vi "Process Data.vi"(7 "AdasLvTemplate in":refnum<class "AdasLvTemplate.lvclass">, 8 "error in":errorcluster, 11 "Node in":refnum<class "BLS Power Supply Template.lvclass">) -> (0 "error out":errorcluster, 3 "Node out":refnum<class "BLS Power Supply Template.lvclass">, 5 "AdasLvTemplate out":refnum<class "AdasLvTemplate.lvclass">)   [LabVIEW 2023, in "BLS Power Supply Template.lvlib" / "BLS Power Supply Template.lvclass"]
uses:
  BLS Power Supply Template.lvclass
  BLS Power Supply Template.lvclass/BLS Power Supply Template.ctl
  bls-capabilities/src/Capabilities/High Level Capabilities/Power Supply/Power Supply.lvclass
  bls-capabilities/src/Capabilities/High Level Capabilities/Power Supply/Voltage Read Single.vi
  bls-capabilities/src/Capabilities/High Level Capabilities/Power Supply/Output Enable Read Single.vi
  bls-capabilities/src/Capabilities/High Level Capabilities/Power Supply/Current Read Single.vi
  bls-capabilities/src/Capabilities/High Level Capabilities/Power Supply/Voltage Max Read Single.vi
  bls-capabilities/src/Capabilities/High Level Capabilities/Power Supply/Voltage Min Read Single.vi
  bls-capabilities/src/Capabilities/High Level Capabilities/Power Supply/Current Max Read Single.vi
  bls-capabilities/src/Capabilities/High Level Capabilities/Power Supply/Current Min Read Single.vi
  bls-capabilities/src/Capabilities/High Level Capabilities/Power Supply/Power Max Read Single.vi
  bls-capabilities/src/Capabilities/High Level Capabilities/Power Supply/Power Min Read Single.vi
  bls-capabilities/src/Capabilities/High Level Capabilities/Power Supply/Voltage Grad Read Single.vi
  bls-capabilities/src/Capabilities/High Level Capabilities/Power Supply/Power Read Single.vi
  bls-capabilities/src/Capabilities/High Level Capabilities/Power Supply/Power Grad Read Single.vi
  bls-capabilities/src/Capabilities/High Level Capabilities/Power Supply/Current Grad Read Single.vi
  bls-capabilities/src/Capabilities/High Level Capabilities/Power Supply/Control Mode Read Single.vi
  bls-capabilities/src/Capabilities/High Level Capabilities/Power Supply/Error Channels Write Single.vi
  bls-capabilities/src/Capabilities/High Level Capabilities/Power Supply/Control Mode Write Single.vi
  bls-capabilities/src/Capabilities/High Level Capabilities/Power Supply/Power Write Single.vi
  bls-capabilities/src/Capabilities/High Level Capabilities/Power Supply/Current Write Single.vi
  bls-capabilities/src/Capabilities/High Level Capabilities/Power Supply/Output Enable Write Single.vi
  bls-capabilities/src/Capabilities/High Level Capabilities/Power Supply/Voltage Write Single.vi
  <vilib>/ADAS Replay HIL/ADAS Plugin Utilities/AdasLvTemplate/AdasLvTemplate.lvclass
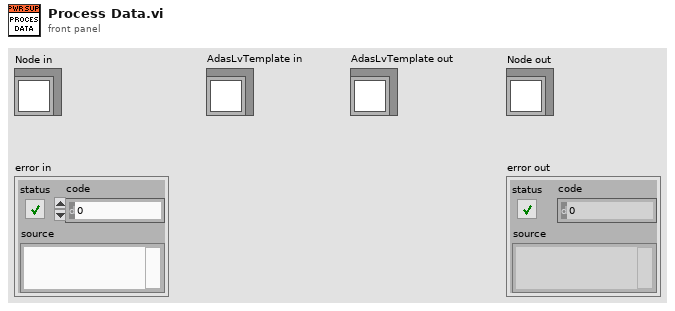
[diagram p1: front panel]
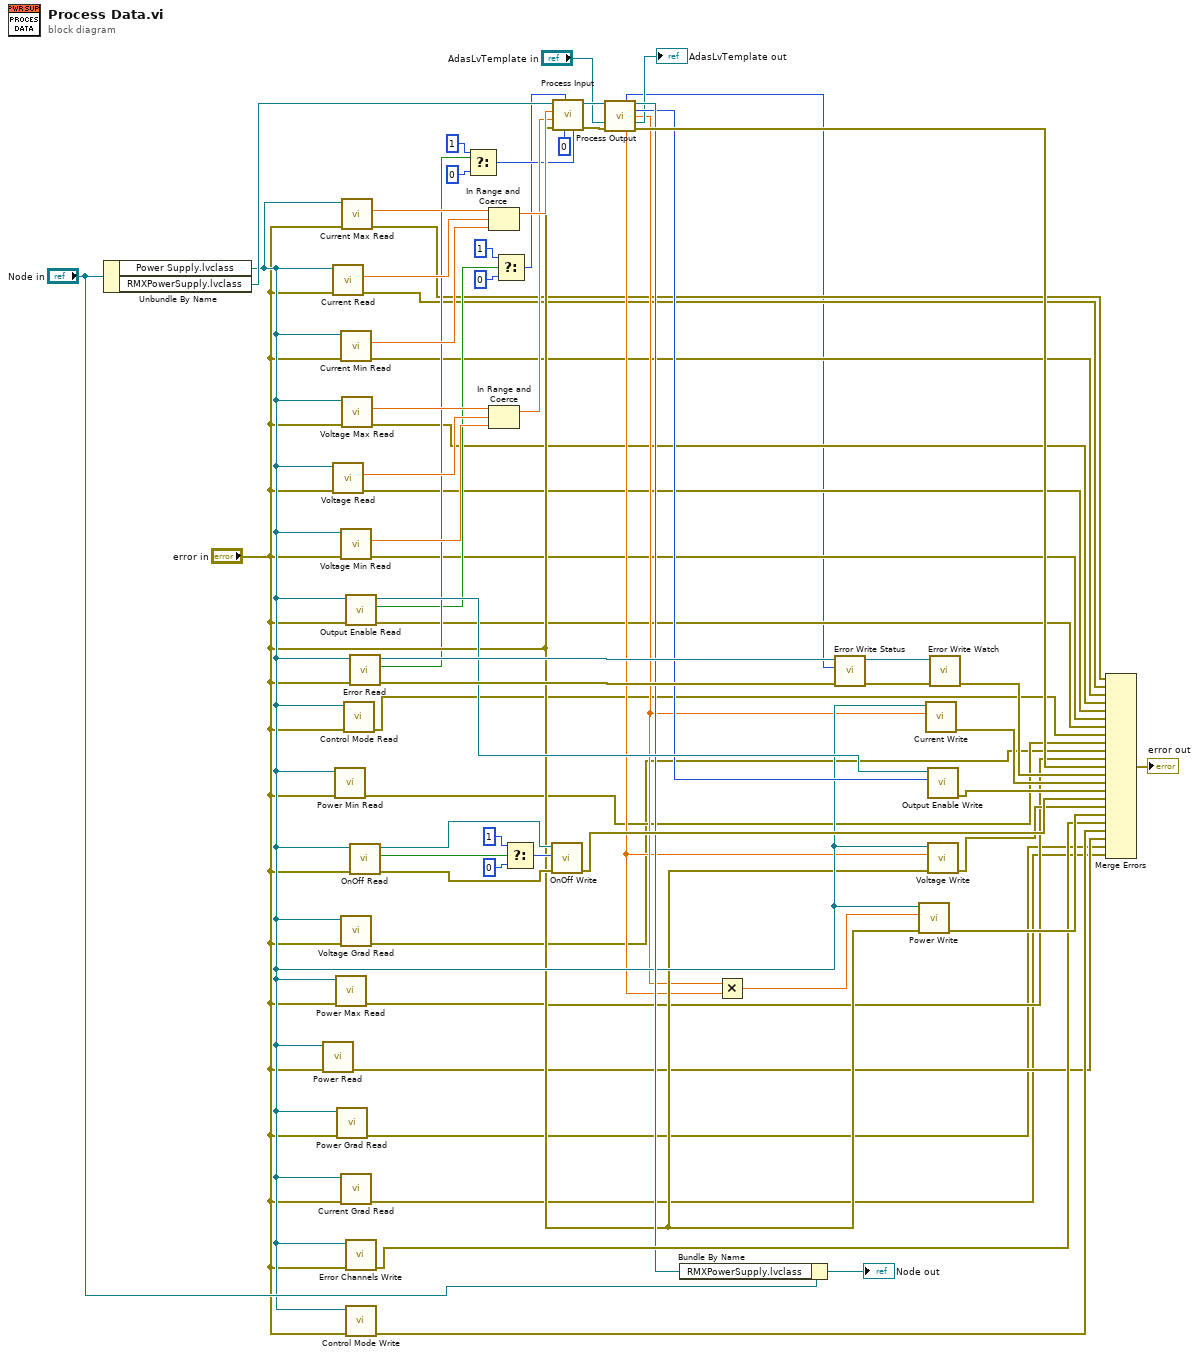
[diagram p0: block diagram]
diagram:
  n1 = Unbundle By Name("Node in") -> ("Power Supply.lvclass"=w28:refnum<class "Power Supply.lvclass">, "RMXPowerSupply.lvclass"=w54:refnum<class "RMXPowerSupply.lvclass">)
  n2 = call-poly "Power Read.vi"("error in"="error in", "Power Supply In"=w28) -> ("error out"=w5:errorcluster)  [unwired: 6 in, 3 out]
  n3 = call-poly "Current Read.vi"("error in"="error in", "Power Supply In"=w28) -> ("error out"=w15:errorcluster, "Current SP"=w38:dbl)  [unwired: 6 in, 2 out]
  n4 = call-poly "Voltage Read.vi"("error in"="error in", "Power Supply In"=w28) -> ("error out"=w12:errorcluster, "Voltage SP"=w43:dbl)  [unwired: 6 in, 2 out]
  n5 = call-poly "Power Min Read.vi"("error in"="error in", "Power Supply In"=w28) -> ("error out"=w8:errorcluster)  [unwired: 6 in, 3 out]
  n6 = call-poly "Power Max Read.vi"("error in"="error in", "Power Supply In"=w28) -> ("error out"=w6:errorcluster)  [unwired: 6 in, 3 out]
  n7 = call-poly "Power Grad Read.vi"("error in"="error in", "Power Supply In"=w28) -> ("error out"=w4:errorcluster)  [unwired: 6 in, 3 out]
  n8 = call-poly "Current Min Read.vi"("error in"="error in", "Power Supply In"=w28) -> ("error out"=w14:errorcluster, "Current Min SP"=w39:dbl)  [unwired: 6 in, 2 out]
  n9 = call-poly "Voltage Min Read.vi"("error in"="error in", "Power Supply In"=w28) -> ("error out"=w11:errorcluster, "Voltage Min SP"=w45:dbl)  [unwired: 6 in, 2 out]
  n10 = call-poly "Voltage Grad Read.vi"("error in"="error in", "Power Supply In"=w28) -> ("error out"=w7:errorcluster)  [unwired: 6 in, 3 out]
  n11 = call-poly "Current Grad Read.vi"("error in"="error in", "Power Supply In"=w28) -> ("error out"=w3:errorcluster)  [unwired: 6 in, 3 out]
  n12 = call-poly "Current Max Read.vi"("error in"="error in", "Power Supply In"=w28) -> ("error out"=w16:errorcluster, "Current Max SP"=w40:dbl)  [unwired: 6 in, 2 out]
  n13 = call-poly "Voltage Max Read.vi"("error in"="error in", "Power Supply In"=w28) -> ("error out"=w13:errorcluster, "Voltage Max SP"=w44:dbl)  [unwired: 6 in, 2 out]
  n14 = call-poly "Control Mode Read.vi"("error in"="error in", "Power Supply In"=w28) -> ("error out"=w9:errorcluster)  [unwired: 6 in, 3 out]
  n15 = call-poly "Output Enable Read.vi"("error in"="error in", "Power Supply In"=w28) -> ("error out"=w10:errorcluster, "Output Enable ACT"=w20:bool, "Power Supply Out"=w35:refnum<class "Power Supply.lvclass">)  [unwired: 6 in, 1 out]
  n16 = call-poly "Error Channels Write.vi"("error in"="error in", "Power Supply In"=w28) -> ("error out"=w58:errorcluster)  [unwired: 8 in, 1 out]
  n17 = call-poly "Control Mode Write.vi"("error in"="error in", "Power Supply In"=w28) -> ("error out"=w57:errorcluster)  [unwired: 8 in, 1 out]
  n18 = call "Error Read.vi"("error in"="error in", "Power Supply In"=w28) -> ("error out"=w42:errorcluster, "Error ACT"=w24:bool, "Power Supply Out"=w41:refnum<class "Power Supply.lvclass">)  [unwired: 6 in, 1 out]
  n19 = call "OnOff Read.vi"("error in"="error in", "Power Supply In"=w28) -> ("error out"=w50:errorcluster, "OnOff ACT"=w48:bool, "Power Supply Out"=w36:refnum<class "Power Supply.lvclass">)  [unwired: 6 in, 1 out]
  n20 = Select(t=1, s=w24, f=0) -> (s? t:f=w23:i32)
  n21 = In Range and Coerce(upper limit=w40, x=w38, lower limit=w39) -> (coerced(x)=w34:dbl)  [unwired: 1 out]
  n22 = In Range and Coerce(upper limit=w44, x=w43, lower limit=w45) -> (coerced(x)=w33:dbl)  [unwired: 1 out]
  n23 = Select(t=1, s=w20, f=0) -> (s? t:f=w19:i32)
  n24 = Select(t=1, s=w48, f=0) -> (s? t:f=w49:i32)
  n25 = call "OnOff Write.vi"("error in"=w50, "OnOff STS"=w49, "Power Supply In"=w36) -> ("error out"=w61:errorcluster)  [unwired: 7 in, 1 out]
  n26 = call "Process Input.vi"("Reset"=w23, "Mode"=0, "Switch Control"=w19, "error in"="error in", "Voltage Setpoint"=w33, "Current Setpoint"=w34, "RMXPowerSupply in"=w54) -> ("error out"=w52:errorcluster, "RMXPowerSupply out"=w53:refnum<class "RMXPowerSupply.lvclass">)  [unwired: 3 in]
  n27 = call "Process Output.vi"("RMXPowerSupply in"=w53, "AdasLvTemplate in"="AdasLvTemplate in", "error in"=w52) -> ("ErrorCode"=w1:i32, "RMXPowerSupply out"=w32:refnum<class "RMXPowerSupply.lvclass">, "Output Status"=w31:i32, "Current"=w18:dbl, "AdasLvTemplate out"=→"AdasLvTemplate out":refnum<class "AdasLvTemplate.lvclass">, "Voltage to Write"=w17:dbl, "error out"=w51:errorcluster)  [unwired: 5 in, 1 out]
  n28 = Bundle By Name(cluster="Node in", "RMXPowerSupply.lvclass"=w32) -> (→"Node out":refnum<class "BLS Power Supply Template.lvclass">)
  n29 = Multiply(x=w18, y=w17) -> (x*y=w37:dbl)
  n30 = call "Error Write Status.vi"("error in"=w42, "Error STS"=w1, "Power Supply In"=w41) -> ("error out"=w66:errorcluster, "Power Supply Out"=w65:refnum<class "Power Supply.lvclass">)  [unwired: 7 in]
  n31 = call-poly "Power Write.vi"("error in"="error in", "Power AV"=w37, "Power Supply In"=w28) -> ("error out"=w59:errorcluster)  [unwired: 7 in, 1 out]
  n32 = call-poly "Current Write.vi"("Current AV"=w18, "Power Supply In"=w28) -> ("error out"=w63:errorcluster)  [unwired: 8 in, 1 out]
  n33 = call-poly "Output Enable Write.vi"("Output Enable STS"=w31, "Power Supply In"=w35) -> ("error out"=w62:errorcluster)  [unwired: 8 in, 1 out]
  n34 = call-poly "Voltage Write.vi"("error in"="error in", "Voltage AV"=w17, "Power Supply In"=w28) -> ("error out"=w60:errorcluster)  [unwired: 7 in, 1 out]
  n35 = call "Error Write Watch.vi"("error in"=w66, "Power Supply In"=w65) -> ("error out"=w64:errorcluster)  [unwired: 8 in, 1 out]
  n36 = Merge Errors(w16, w15, w14, w13, w12, w11, w10, w9, w8, w7, w6, w51, w64, w63, w62, w61, w60, w59, w58, w57, w5, w4, w3) -> (→"error out":errorcluster)
